vi "PASCO_PID.vi"(0 "Desired Rate":dbl(slide) scale=-1.0..1.0, 5 "Actual Rate":dbl, 9 "Integral Reset":bool, 12 "P Gain":dbl=1.0, 13 "I Gain":dbl=0.01, 14 "D Gain":dbl) -> (4 "PWM Power":dbl)   [LabVIEW 2012]
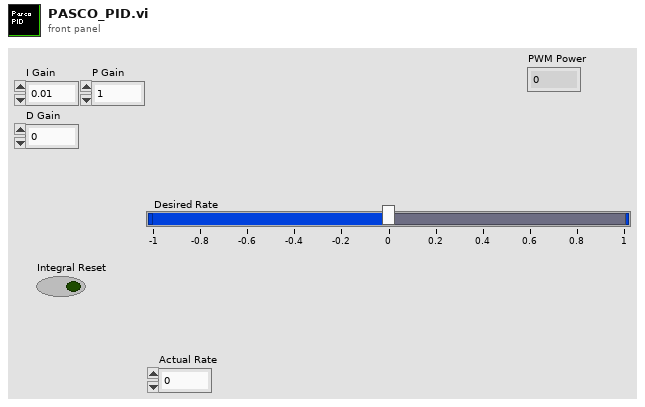
[diagram p1: front panel]
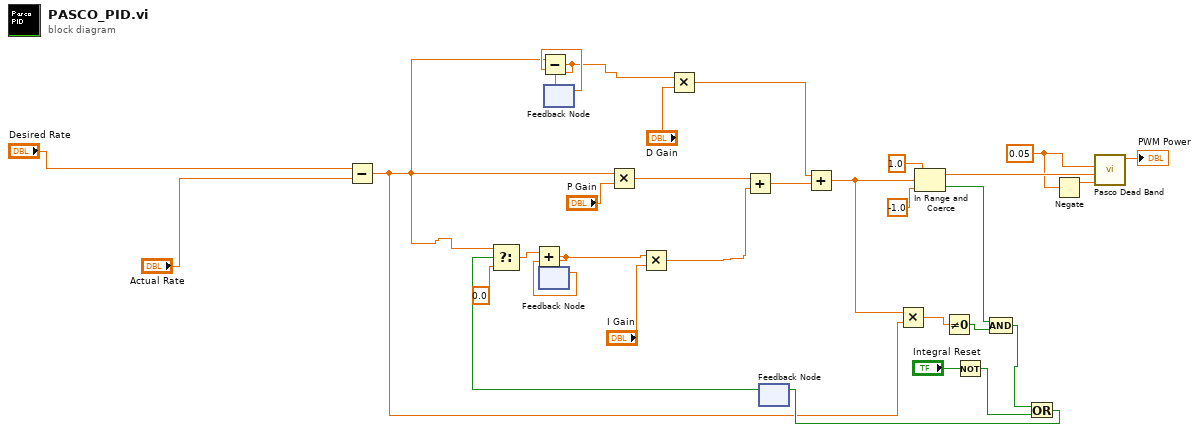
[diagram p0: block diagram]
diagram:
  w17 = 0.05 ("upper limit")
  n1 = Subtract(x="Desired Rate", y="Actual Rate") -> (x-y=w5:dbl)
  n2 = feedback #1() -> (w2:dbl)  [unwired: 1 in]
  n3 = feedback #2() -> (w28:dbl)  [unwired: 1 in]
  n4 = Subtract(x=w5, y=w28) -> (x-y=w3:dbl)
  n5 = feedback-in #2(w3) -> ()
  n6 = Multiply(x=w5, y="P Gain") -> (x*y=w14:dbl)
  n7 = Multiply(x=w3, y="D Gain") -> (x*y=w4:dbl)
  n8 = feedback #3() -> (w16:bool)  [unwired: 1 in]
  n9 = Select(t=w5, s=w16, f=0.0) -> (s? t:f=w22:dbl)
  n10 = Add(x=w22, y=w2) -> (x+y=w1:dbl)
  n11 = feedback-in #1(w1) -> ()
  n12 = Multiply(x=w1, y="I Gain") -> (x*y=w6:dbl)
  n13 = Add(x=w14, y=w6) -> (x+y=w21:dbl)
  n14 = Add(x=w4, y=w21) -> (x+y=w20:dbl)
  n15 = Multiply(x=w20, y=w5) -> (x*y=w26:dbl)
  n16 = In Range and Coerce(upper limit=1.0, x=w20, lower limit=-1.0) -> (coerced(x)=w19:dbl, In Range?=w24:bool)
  n17 = Not Equal To 0?(x=w26) -> (x != 0?=w25:bool)
  n18 = Not(x="Integral Reset") -> (.not. x?=w9:bool)
  n19 = Compound Arithmetic op=AND(w24, w25) -> (w10:bool)
  n20 = Or(x=w10, y=w9) -> (x .or. y?=w8:bool)
  n21 = feedback-in #3(w8) -> ()
  n22 = Negate(x=w17) -> (-x=w18:dbl)
  n23 = call "Pasco Dead Band.vi"("lower limit"=w18, "PWM Power"=w19, "upper limit"=w17) -> ("PWM Power"=→"PWM Power":dbl)  [unwired: 7 in, 1 out]
